vi "Send ACK Msg.vi"(7 "Enable?":bool, 8 "error in (no error)":errorcluster, 9 "Index":u32, 10 "Message":string, 11 "HAL  in":refnum<queue>) -> (0 "error out":errorcluster, 1 "dup Index":u32, 3 "HAL  out":refnum<queue>)   [LabVIEW 2014, in "HWAsyncLoop.lvlib"]
uses:
  HWAsyncLoop.lvlib
  APIs/Message Queue/Message Cluster.ctl
  APIs/Message Queue/Enqueue Message (Single).vi
  APIs/Message Queue/WINFAS 2 Message Queue.lvlib
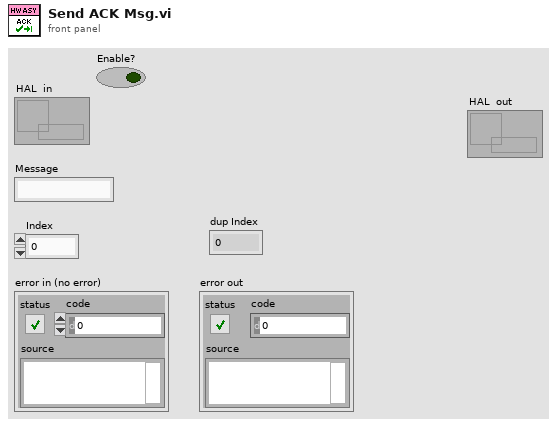
[diagram p1: front panel]
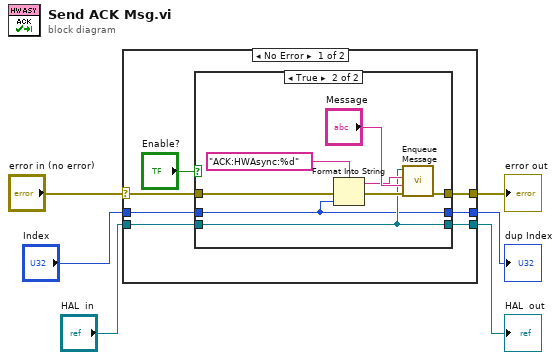
[diagram p0: block diagram]
diagram:
  n1 = case shown="No Error" "error in (no error)" {
    selector: "error in (no error)" -> [w12 w27]
    tunnel: [w13 w27] -> w6
    tunnel: "HAL  in" -> [w10 w26]
    tunnel: [w9 w26] -> w3
    tunnel: "Index" -> [w8 w25]
    tunnel: [w7 w25] -> w1
    frame No Error {
      n2 = case shown="True" "Enable?" {
        tunnel: [w16 w24] -> w13
        tunnel: w12 -> [w16 w20]
        tunnel: w10 -> [w15 w18]
        tunnel: [w15 w18] -> w9
        tunnel: w8 -> [w14 w17]
        tunnel: [w14 w17] -> w7
        frame False {
        }
        frame True {
          n3 = Format Into String(format string="ACK:HWAsync:%d" ("Message"), error in=w20, w17) -> (resulting string=w21:string, error out=w19:errorcluster)  [unwired: 1 in]
          n4 = call-poly "Enqueue Message.vi"("error in (no error)"=w19, "Message Data"="Message", "Message"=w21, "Message Queue"=w18) -> ("error out"=w24:errorcluster)  [unwired: 6 in, 1 out]
        }
      }
    }
    frame Error {
    }
  }
  "error out" <- w6
  "HAL  out" <- w3
  "dup Index" <- w1
